vi "BIB Board Number (SubVI).vi"(11 "JSON string":string) -> (0 "ROperationStatus":string[](array[string]), 3 "LOperationStatus":string[](array[string]))   [LabVIEW 2017]
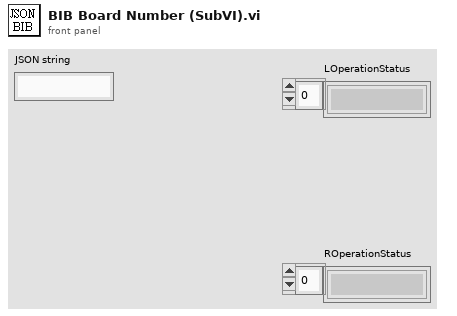
[diagram p1: front panel]
types:
  T1 = cluster{"LBoardNumber":string, "RBoardNumber":string}
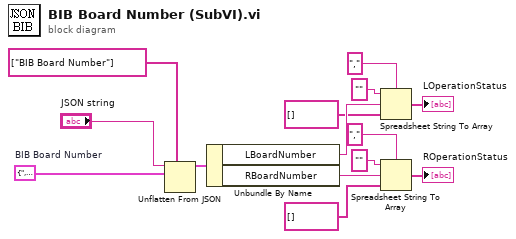
[diagram p0: block diagram]
diagram:
  w12 = T1 {"LBoardNumber"=",,,,,,,,,,,,,,,,,,,,,,,,,", "RBoardNumber"=",,,,,,,,,,,,,,,,,,,,,,,,,"}  # BIB Board Number
  n1 = Unflatten From JSON(path=string[] ["BIB Board Number"], JSON string="JSON string", type and defaults=w12) -> (value=w1:T1)  [unwired: 4 in, 1 out]
  n2 = Unbundle By Name(w1) -> ("LBoardNumber"=w6:string, "RBoardNumber"=w11:string)
  n3 = Spreadsheet String To Array(delimiter (Tab)=",", format string="", spreadsheet string=w6, array type (2D Dbl)=string[] []) -> (array=→"LOperationStatus":string[])
  n4 = Spreadsheet String To Array(delimiter (Tab)=",", format string="", spreadsheet string=w11, array type (2D Dbl)=string[] []) -> (array=→"ROperationStatus":string[])
